vi "Quaternion_Get_W.vi"(11 "Quaternion":T1={"R"=1.0, "V"=[0.0, 0.0, 0.0]}) -> (3 "W":dbl=1.0)   [LabVIEW 2019, in "Trajectory_Library.lvlib"]
doc: "Return the W component of the quaternion\n\nParameters:\n - Quaternion -- The quaternion data cluster. \n\nReturns:\n - W - Returns W component of the quaternion."
uses:
  Trajectory_Library.lvlib
  TypeDef/QUATERNION.ctl
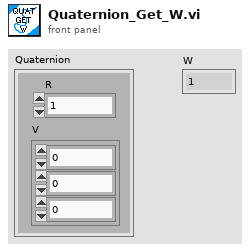
[diagram p1: front panel]
types:
  T1 = typedef "Trajectory_Library.lvlib/QUATERNION.ctl" = cluster{"R":dbl, "V":dbl[]}
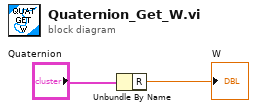
[diagram p0: block diagram]
diagram:
  n1 = Unbundle By Name("Quaternion") -> ("R"=→"W":dbl)
